vi "test Add Analog Replay Returns Successfully.vi"(8 "error in (no error)":errorcluster, 11 "TestCase in":refnum<class "Scripting API Test Case.lvclass">) -> (0 "error out":errorcluster, 3 "TestCase out":refnum<class "Scripting API Test Case.lvclass">)   [LabVIEW 2015, in "Scripting API Test Case.lvclass"]
uses:
  Scripting API Test Case.lvclass
  SysDef API/Engine Simulation Toolkit Custom Device Settings.ctl
  <vilib>/NI Veristand/Custom Device API/Custom Device Timed Loop Priority.ctl
  SysDef API/Analog Replay Settings.ctl
  SysDef API/Analog Replay Data Options.ctl
  System Explorer/FPGA Mem Size.ctl
  System Explorer/Position Reference.ctl
  System Explorer/Data Replay Data Selection Method.ctl
  NationalInstruments.VeriStand.SystemDefinitionAPI
  <userlib>/_OpenG.lib/file/file.llb/Append Path to Root if Relative - Scalar__ogtk.vi
  <vilib>/addons/_JKI Toolkits/VI Tester/TestCase.llb/TestCase.lvclass
  SysDef API/Engine Simulation Toolkit SysDef API.lvlib
  <vilib>/NI VeriStand/Custom Device API/Custom Device API.lvlib
  niveristand-custom-device-testing-tools/VeriStandTestUtilities/VeriStandTestUtilities.lvlib
  System Explorer/Engine Simulation Toolkit System Explorer.lvlib
panel:
  out "string":string
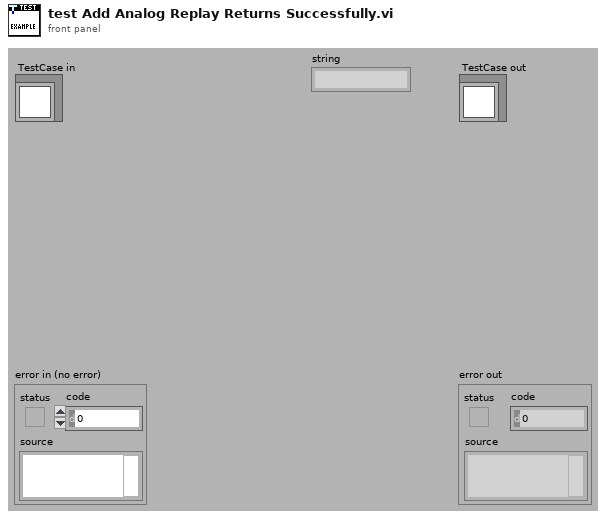
[diagram p1: front panel]
types:
  T1 = typedef "Engine Simulation Toolkit SysDef API.lvlib/Analog Replay Data Options.ctl" = cluster{"Input file":path, "Group":string, "Channel":string, "Reverse":bool, "FPGA Memory Size":T2, "Position reference":T3, "Data selection method":T4, "Offset":i32, "Samples":i32, "Missing teeth location":dbl, "DataPlugin":string}
  T2 = typedef "Engine Simulation Toolkit System Explorer.lvlib/FPGA Mem Size.ctl" = enum16{"65,536", "32,768", "16,384", "8,192", "4,096", "2,048", "1,024"}
  T3 = typedef "Engine Simulation Toolkit System Explorer.lvlib/Position Reference.ctl" = enum16{"Crank angle", "Cycle angle"}
  T4 = typedef "Engine Simulation Toolkit System Explorer.lvlib/Data Replay Data Selection Method.ctl" = enum32{"Manual", "AutoVRCrank"}
  T5 = typedef "Engine Simulation Toolkit SysDef API.lvlib/Analog Replay Settings.ctl" = cluster{"Name":string, "DAC bipolar range (V)":dbl, "Voltage below min speed":dbl, "Min speed (RPM)":dbl, "Voltage at min speed":dbl, "Max speed (RPM)":dbl, "Voltage at max speed":dbl, "Negate playback voltage values at negative engine speed":bool, "Allow run-time override of voltage scaling":bool}
  T6 = typedef "Engine Simulation Toolkit SysDef API.lvlib/Engine Simulation Toolkit Custom Device Settings.ctl" = cluster{"Name":string, "Execution priority":T7, "Rate decimation":i32, "CPU":i32, "Device address":string, "Bitfile path":path, "APUs":string[]}
  T7 = typedef "Custom Device API.lvlib/Custom Device Timed Loop Priority.ctl" = enum32{"Low", "Medium", "High"}
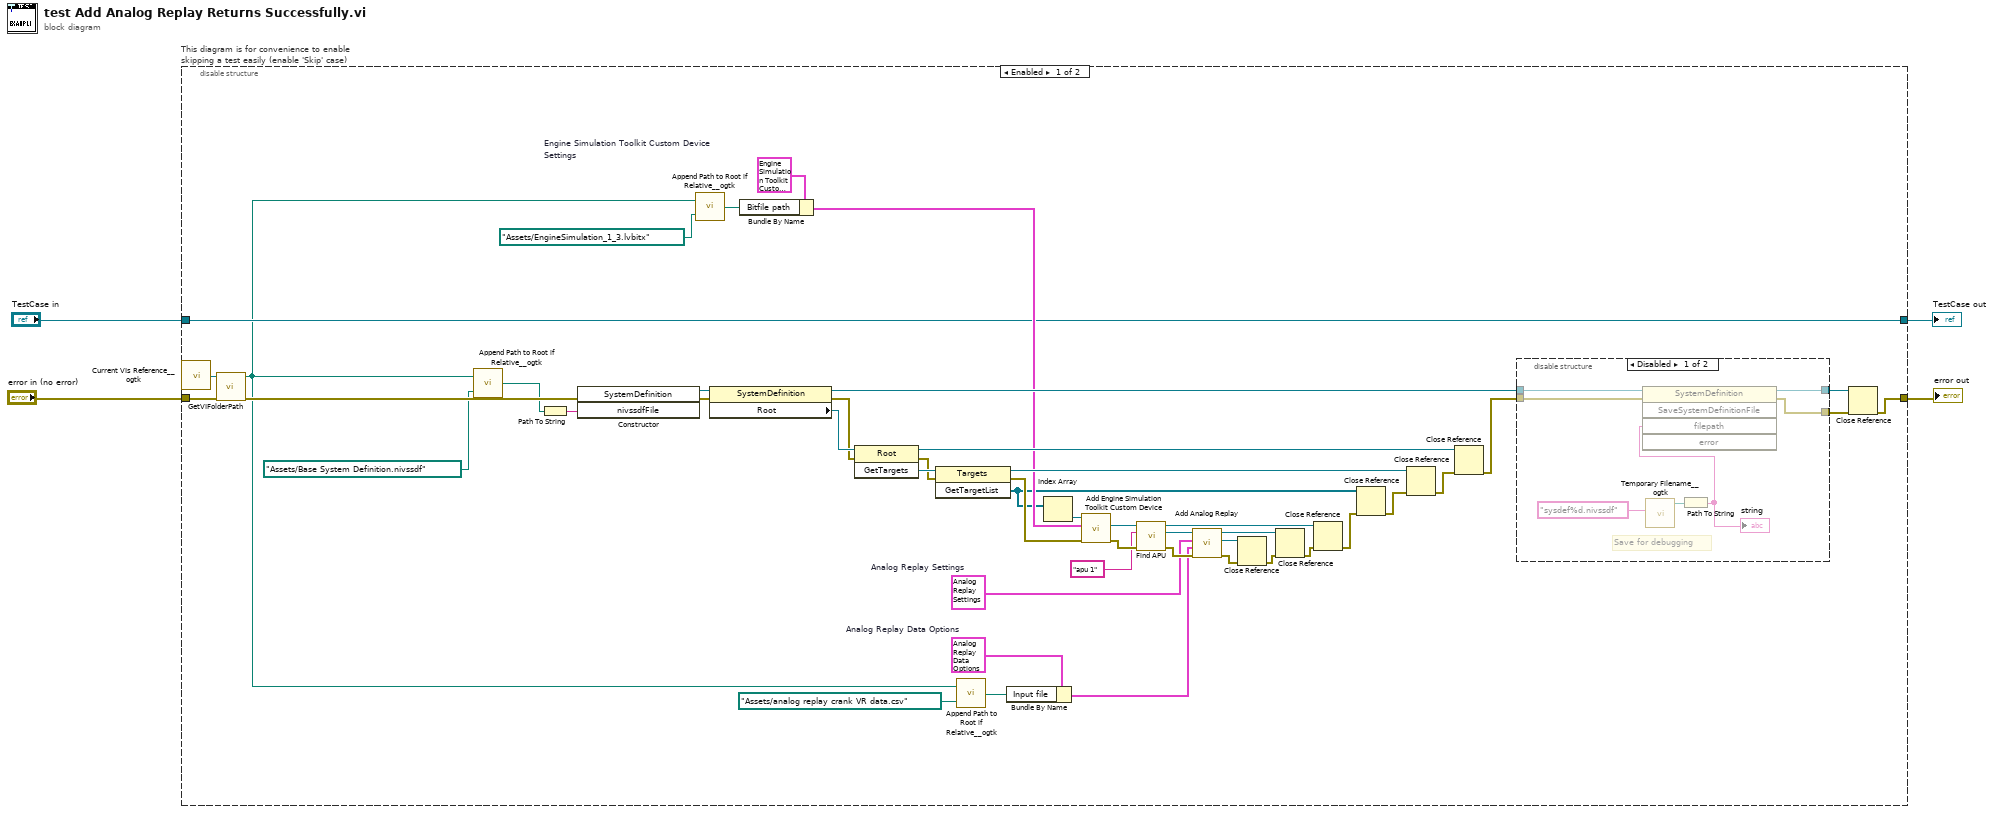
[diagram p0: block diagram]
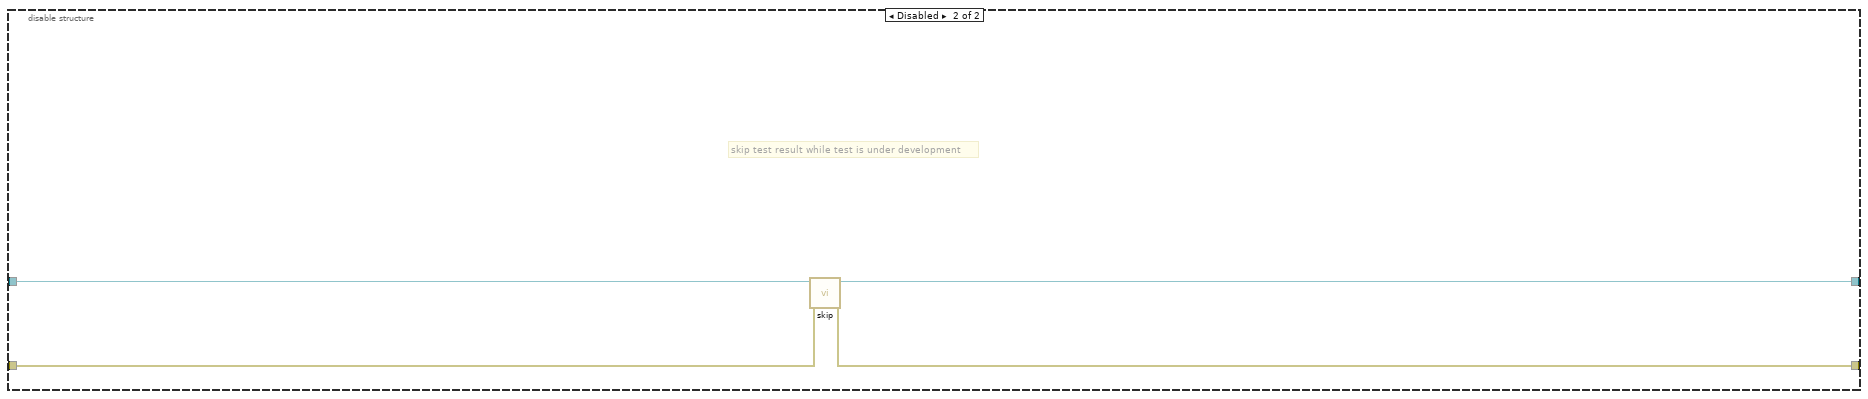
[diagram p3: hidden frame]
diagram:
  n1 = disable-structure "This diagram is for convenience to enable skipping a test easily (enable 'Skip' case)" shown="Enabled" {
    disable-tunnel: "TestCase in" -> [w22 w64]
    disable-tunnel: [w22 w62] -> w1
    disable-tunnel: [w43 w63] -> w3
    disable-tunnel: "error in (no error)" -> [w29 w61]
    frame Enabled {
      w16 = T1 {"Input file"=path "", "Group"="analog replay crank VR data", "Channel"="Ch0", "Reverse"=FALSE, "FPGA Memory Size"=enum."16,384", "Position reference"=enum."Crank angle", "Data selection method"=enum."Manual", "Offset"=0, "Samples"=100000, "Missing teeth location"=0.0, "DataPlugin"="CSV"}  # Analog Replay Data Options
      w17 = T5 {"Name"="replay AO 0", "DAC bipolar range (V)"=10.0, "Voltage below min speed"=0.0, "Min speed (RPM)"=0.0, "Voltage at min speed"=0.0, "Max speed (RPM)"=10000.0, "Voltage at max speed"=10.0, "Negate playback voltage values at negative engine speed"=TRUE, "Allow run-time override of voltage scaling"=FALSE}  # Analog Replay Settings
      w45 = T6 {"Name"="Engine Simulation Toolkit", "Execution priority"=enum."Medium", "Rate decimation"=1, "CPU"=-2, "Device address"="RIO 0", "Bitfile path"=path "", "APUs"=[]}  # Engine Simulation Toolkit Custom Device Settings
      n2 = call <userlib>:"Current VIs Reference__ogtk.vi"() -> ("Current VI's reference"=w30:refnum<vi>)  [unwired: 5 in]
      n3 = call "GetVIFolderPath.vi"("error in (no error)"=w29, "VI Reference in"=w30) -> ("error out"=w28:errorcluster, "VI Folder Path out"=w12:path)  [unwired: 8 in]
      n4 = call-poly <userlib>:"Append Path to Root if Relative__ogtk.vi"("Absolute or Relative Path"=path "Assets/Base System Definition.nivssdf", "Root Path"=w12) -> ("Absolute or Appended Path"=w26:path)
      n5 = Path To String(path=w26) -> (string=w31:string)
      n6 = constructor class="SystemDefinition"(error in=w28, "nivssdfFile"=w31) -> (reference out=w51:refnum<k24>, error out=w50:errorcluster)  [unwired: 2 in, 2 out]
      n7 = call-poly <userlib>:"Append Path to Root if Relative__ogtk.vi"("Absolute or Relative Path"=path "Assets/EngineSimulation_1_3.lvbitx", "Root Path"=w12) -> ("Absolute or Appended Path"=w32:path)
      n8 = property class="SystemDefinition"(reference=w51, error in=w50) -> (reference out=w44:refnum<k24>, error out=w46:errorcluster, "Root"=w49:refnum<k24>)
      n9 = Bundle By Name(cluster=w45, "Bitfile path"=w32) -> (w34:T6)
      n10 = invoke class="Root" method="GetTargets"(reference=w49, error in=w46) -> (reference out=w39:refnum<k24>, error out=w47:errorcluster, "GetTargets"=w48:refnum<k24>)  [unwired: 1 in]
      n11 = invoke class="Targets" method="GetTargetList"(reference=w48, error in=w47) -> (reference out=w38:refnum<k24>, error out=w35:errorcluster, "GetTargetList"=w23:refnum<k24>[])  [unwired: 1 in]
      n12 = call-poly <userlib>:"Append Path to Root if Relative__ogtk.vi"("Absolute or Relative Path"=path "Assets/analog replay crank VR data.csv", "Root Path"=w12) -> ("Absolute or Appended Path"=w14:path)
      n13 = Bundle By Name(cluster=w16, "Input file"=w14) -> (w15:T1)
      n14 = Index Array(array=w23) -> (element=w25:refnum<k24>)  [unwired: 1 in]
      n15 = call "Add Engine Simulation Toolkit Custom Device.vi"("error in (no error)"=w35, "Engine Simulation Toolkit Custom Device Settings"=w34, "Target in"=w25) -> ("error out"=w20:errorcluster, "EST Custom Device"=w21:refnum<k24>)  [unwired: 6 in, 1 out]
      n16 = call "Find APU.vi"("error in (no error)"=w20, "APU name"="apu 1", "EST custom device in"=w21) -> ("error out"=w19:errorcluster, "APU Node"=w18:refnum<k24>, "EST custom device out"=w11:refnum<k24>)  [unwired: 6 in]
      n17 = call "Add Analog Replay.vi"("error in (no error)"=w19, "Analog Replay Data Options"=w15, "Analog Replay Settings"=w17, "APU Node in"=w18) -> ("error out"=w6:errorcluster, "Analog Replay out"=w7:refnum<k24>, "APU Node out"=w8:refnum<k24>)  [unwired: 5 in]
      n18 = Close Reference(reference=w7, error in (no error)=w6) -> (error out=w5:errorcluster)
      n19 = Close Reference(reference=w8, error in (no error)=w5) -> (error out=w9:errorcluster)
      n20 = Close Reference(reference=w11, error in (no error)=w9) -> (error out=w24:errorcluster)
      n21 = Close Reference(reference=w23, error in (no error)=w24) -> (error out=w36:errorcluster)
      n22 = Close Reference(reference=w38, error in (no error)=w36) -> (error out=w37:errorcluster)
      n23 = Close Reference(reference=w39, error in (no error)=w37) -> (error out=w40:errorcluster)
      n24 = disable-structure shown="Disabled" {
        disable-tunnel: w44 -> [w58 w59]
        disable-tunnel: [w57 w60] -> w42
        disable-tunnel: [w56 w59] -> w41
        disable-tunnel: w40 -> [w55 w60]
        frame Disabled {
          # "Save for debugging"
          n25 = call <userlib>:"Temporary Filename__ogtk.vi"("pattern (lvtemp%d.tmp)"="sysdef%d.nivssdf") -> ("file in tmp dir"=w53:path)  [unwired: 5 in, 1 out]
          n26 = Path To String(path=w53) -> (string=w52:string)
          "string" <- w52
          n27 = invoke class="SystemDefinition" method="SaveSystemDefinitionFile"(reference=w58, error in=w55, "filepath"=w52) -> (reference out=w56:refnum<k24>, error out=w57:errorcluster)  [unwired: 2 in, 3 out]
        }
        frame Enabled {
        }
      }
      n28 = Close Reference(reference=w41, error in (no error)=w42) -> (error out=w43:errorcluster)
    }
    frame Disabled {
      # "skip test result while test is under development"
      n29 = call <vilib>:"skip.vi"("error in (no error)"=w61, "TestCase in"=w64) -> ("error out"=w63:errorcluster, "TestCase out"=w62:refnum<class "Scripting API Test Case.lvclass">)  [unwired: 8 in]
    }
  }
  "error out" <- w3
  "TestCase out" <- w1
